vi "target_exists.vi"(8 "error in":errorcluster, 10 "Target Name":string, 11 "vsd reference":refnum<k24>) -> (0 "error out":errorcluster, 1 "target if exists":refnum<k24>, 2 "Target Exists":bool, 3 "vsd reference out":refnum<k24>)   [LabVIEW 2020]
uses:
  NationalInstruments.VeriStand.SystemDefinitionAPI
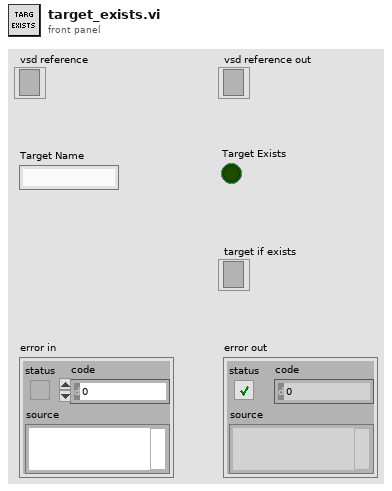
[diagram p1: front panel]
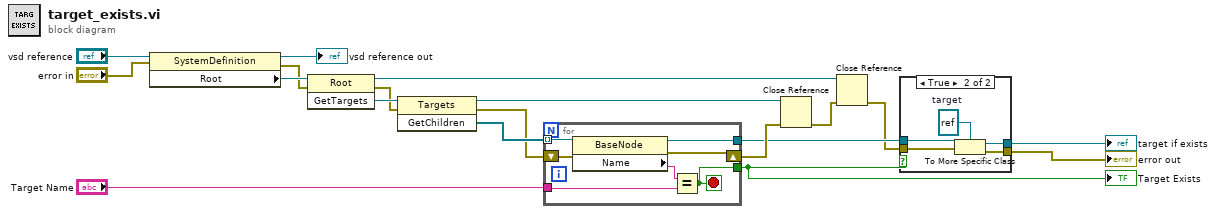
[diagram p0: block diagram]
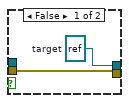
[diagram p2: hidden frame]
diagram:
  n1 = property class="SystemDefinition"(reference="vsd reference", error in="error in") -> (reference out=→"vsd reference out":refnum<k24>, error out=w17:errorcluster, "Root"=w19:refnum<k24>)
  n2 = invoke class="Root" method="GetTargets"(reference=w19, error in=w17) -> (reference out=w11:refnum<k24>, error out=w6:errorcluster, "GetTargets"=w14:refnum<k24>)  [unwired: 1 in]
  n3 = invoke class="Targets" method="GetChildren"(reference=w14, error in=w6) -> (reference out=w10:refnum<k24>, error out=w12:errorcluster, "GetChildren"=w13:refnum<k24>[])  [unwired: 1 in]
  n4 = for {
    tunnel: w13 -> [w26] mode=indexing
    shift-right: [w24] -> w9
    shift-left: w12 -> [w25]
    tunnel: "Target Name" -> [w22]
    tunnel: [w21] -> w5
    tunnel: [w20] -> w2
    stop <- w20 stop-if-true
    n5 = property class="BaseNode"(reference=w26, error in=w25) -> (reference out=w21:refnum<k24>, error out=w24:errorcluster, "Name"=w23:string)
    n6 = Equal?(x=w23, y=w22) -> (x = y?=w20:bool)
  }
  "Target Exists" <- w2
  n7 = Close Reference(reference=w10, error in (no error)=w9) -> (error out=w8:errorcluster)
  n8 = Close Reference(reference=w11, error in (no error)=w8) -> (error out=w4:errorcluster)
  n9 = case shown="True" w2 {
    tunnel: w5 -> [_ w33]
    tunnel: w4 -> [w28 w31]
    tunnel: [w27 w30] -> w1
    tunnel: [w28 w29] -> w3
    frame False {
      w27 = refnum<k24> refnum  # target
    }
    frame True {
      w32 = refnum<k24> refnum  # target
      n10 = To More Specific Class(target class=w32, reference=w33, error in=w31) -> (specific class reference=w30:refnum<k24>, error out=w29:errorcluster)
    }
  }
  "error out" <- w3
  "target if exists" <- w1
